vi "test-ltv-unicycle-controller-Test2.vi"() -> (3 "All tests passed":bool)   [LabVIEW 2019]
uses:
  <vilib>/Rock Robotics/WPI/ThirdParty/JAS_Junk/TrajLib/Trajectory_Library.lvlib
  <vilib>/Rock Robotics/WPI/ThirdParty/JAS_Junk/TrajLib/Enum/TRAJECTORY_SPLINE_TYPE_ENUM.ctl
  <vilib>/numeric/Random Number (Range) DBL.vi
  <vilib>/Rock Robotics/WPI/ThirdParty/JAS_Junk/TrajLib/TypeDef/TRANSLATION2D.ctl
  <vilib>/Rock Robotics/WPI/ThirdParty/JAS_Junk/TrajLib/TypeDef/ROTATION2D.ctl
  <vilib>/Rock Robotics/WPI/ThirdParty/JAS_Junk/TrajLib/TypeDef/POSE2D.ctl
  <vilib>/Rock Robotics/WPI/ThirdParty/JAS_Junk/TrajLib/TypeDef/TRAJ_STATE.ctl
  <vilib>/Rock Robotics/WPI/ThirdParty/JAS_Junk/TrajLib/TypeDef/TRAJECTORY.ctl
  <vilib>/Rock Robotics/WPI/ThirdParty/JAS_Junk/TrajLib/TypeDef/CHASSIS_SPEEDS.ctl
  <vilib>/Rock Robotics/WPI/ThirdParty/JAS_Junk/TrajLib/TypeDef/LTV_UNICYCLE_CONTROLLER.ctl
  <vilib>/Rock Robotics/WPI/ThirdParty/JAS_Junk/TrajLib/TypeDef/FUNCTION_GENERATOR_MATRIX.ctl
panel:
  in  "Use Rate Limit":bool=TRUE
  in  "Use Noise":bool
  out "Any Calc Error":bool
  out "At Reference":bool
  out "Waveform Graph":dbl[][](graph)
  out "Ctrl":T1={"States"=0, "Inputs"=0, "PoseError"={"TRANSLATION"={"X"=0.0, "Y"=0.0}, "ROTATION"={"VALUE"=0.0, "COS"=1.0, "SIN"=0.0}}, "PoseTolerance"={"TRANSLATION"={"X"=0.0, "Y"=0.0}, "ROTATION"={"VALUE"=0.0, "COS"=1.0, "SIN"=0.0}}, "Dt"=0.02, "Enabled"=FALSE, "LQR_K_Table"={"Table Xs"=[], "Table Ys"=[], "MinX"=0.0, "MaxX"=0.0, "ItemCount"=0, "Rows"=0, "Columns"=0}} {"PoseTolerance"."ROTATION"."SIN" format="%13.4f"; "PoseTolerance"."ROTATION"."COS" format="%13.4f"; "PoseTolerance"."ROTATION"."VALUE" format="%13.4f"; "PoseTolerance"."TRANSLATION"."Y" format="%14.3f"; "PoseTolerance"."TRANSLATION"."X" format="%14.3f"; "PoseError"."ROTATION"."SIN" format="%13.4f"; "PoseError"."ROTATION"."COS" format="%13.4f"; "PoseError"."ROTATION"."VALUE" format="%13.4f"; "PoseError"."TRANSLATION"."Y" format="%14.3f"; "PoseError"."TRANSLATION"."X" format="%14.3f"}
  out "ChassisSpeeds":T6 {"vOmega" format="%10.3f"; "vY" format="%10.3f"; "vX" format="%10.3f"}
  out "XY Graph":cluster{dbl[], dbl[]}[](graph)
  out "X":bool
  out "Y":bool
  out "Rot":bool
  out "TotalTime_Sec":dbl
  out "OutputTRAJ_STATE":T7={"TimeSeconds"=0.0, "Velocity"=0.0, "Acceleration"=0.0, "POSE"={"TRANSLATION"={"X"=0.0, "Y"=0.0}, "ROTATION"={"VALUE"=0.0, "COS"=1.0, "SIN"=0.0}}, "Curvature"=0.0} {"POSE"."ROTATION"."SIN" format="%13.4f"; "POSE"."ROTATION"."COS" format="%13.4f"; "POSE"."ROTATION"."VALUE" format="%13.4f"; "POSE"."TRANSLATION"."Y" format="%14.3f"; "POSE"."TRANSLATION"."X" format="%14.3f"}
  out "UpdatedPose":T2 {"ROTATION"."SIN" format="%13.4f"; "ROTATION"."COS" format="%13.4f"; "ROTATION"."VALUE" format="%13.4f"; "TRANSLATION"."Y" format="%14.3f"; "TRANSLATION"."X" format="%14.3f"}
  out "TrajStatePose":T2={"TRANSLATION"={"X"=0.0, "Y"=0.0}, "ROTATION"={"VALUE"=0.0, "COS"=1.0, "SIN"=0.0}} {"ROTATION"."SIN" format="%13.4f"; "ROTATION"."COS" format="%13.4f"; "ROTATION"."VALUE" format="%13.4f"; "TRANSLATION"."Y" format="%14.3f"; "TRANSLATION"."X" format="%14.3f"}
  out "Calc Error":bool
  out "Create\nError":bool
  out "TRAJECTORY":T8 {"States"."POSE"."ROTATION"."SIN" format="%13.4f"; "States"."POSE"."ROTATION"."COS" format="%13.4f"; "States"."POSE"."ROTATION"."VALUE" format="%13.4f"; "States"."POSE"."TRANSLATION"."Y" format="%14.3f"; "States"."POSE"."TRANSLATION"."X" format="%14.3f"; "TotalTImeSecs" format="%20.3f"}
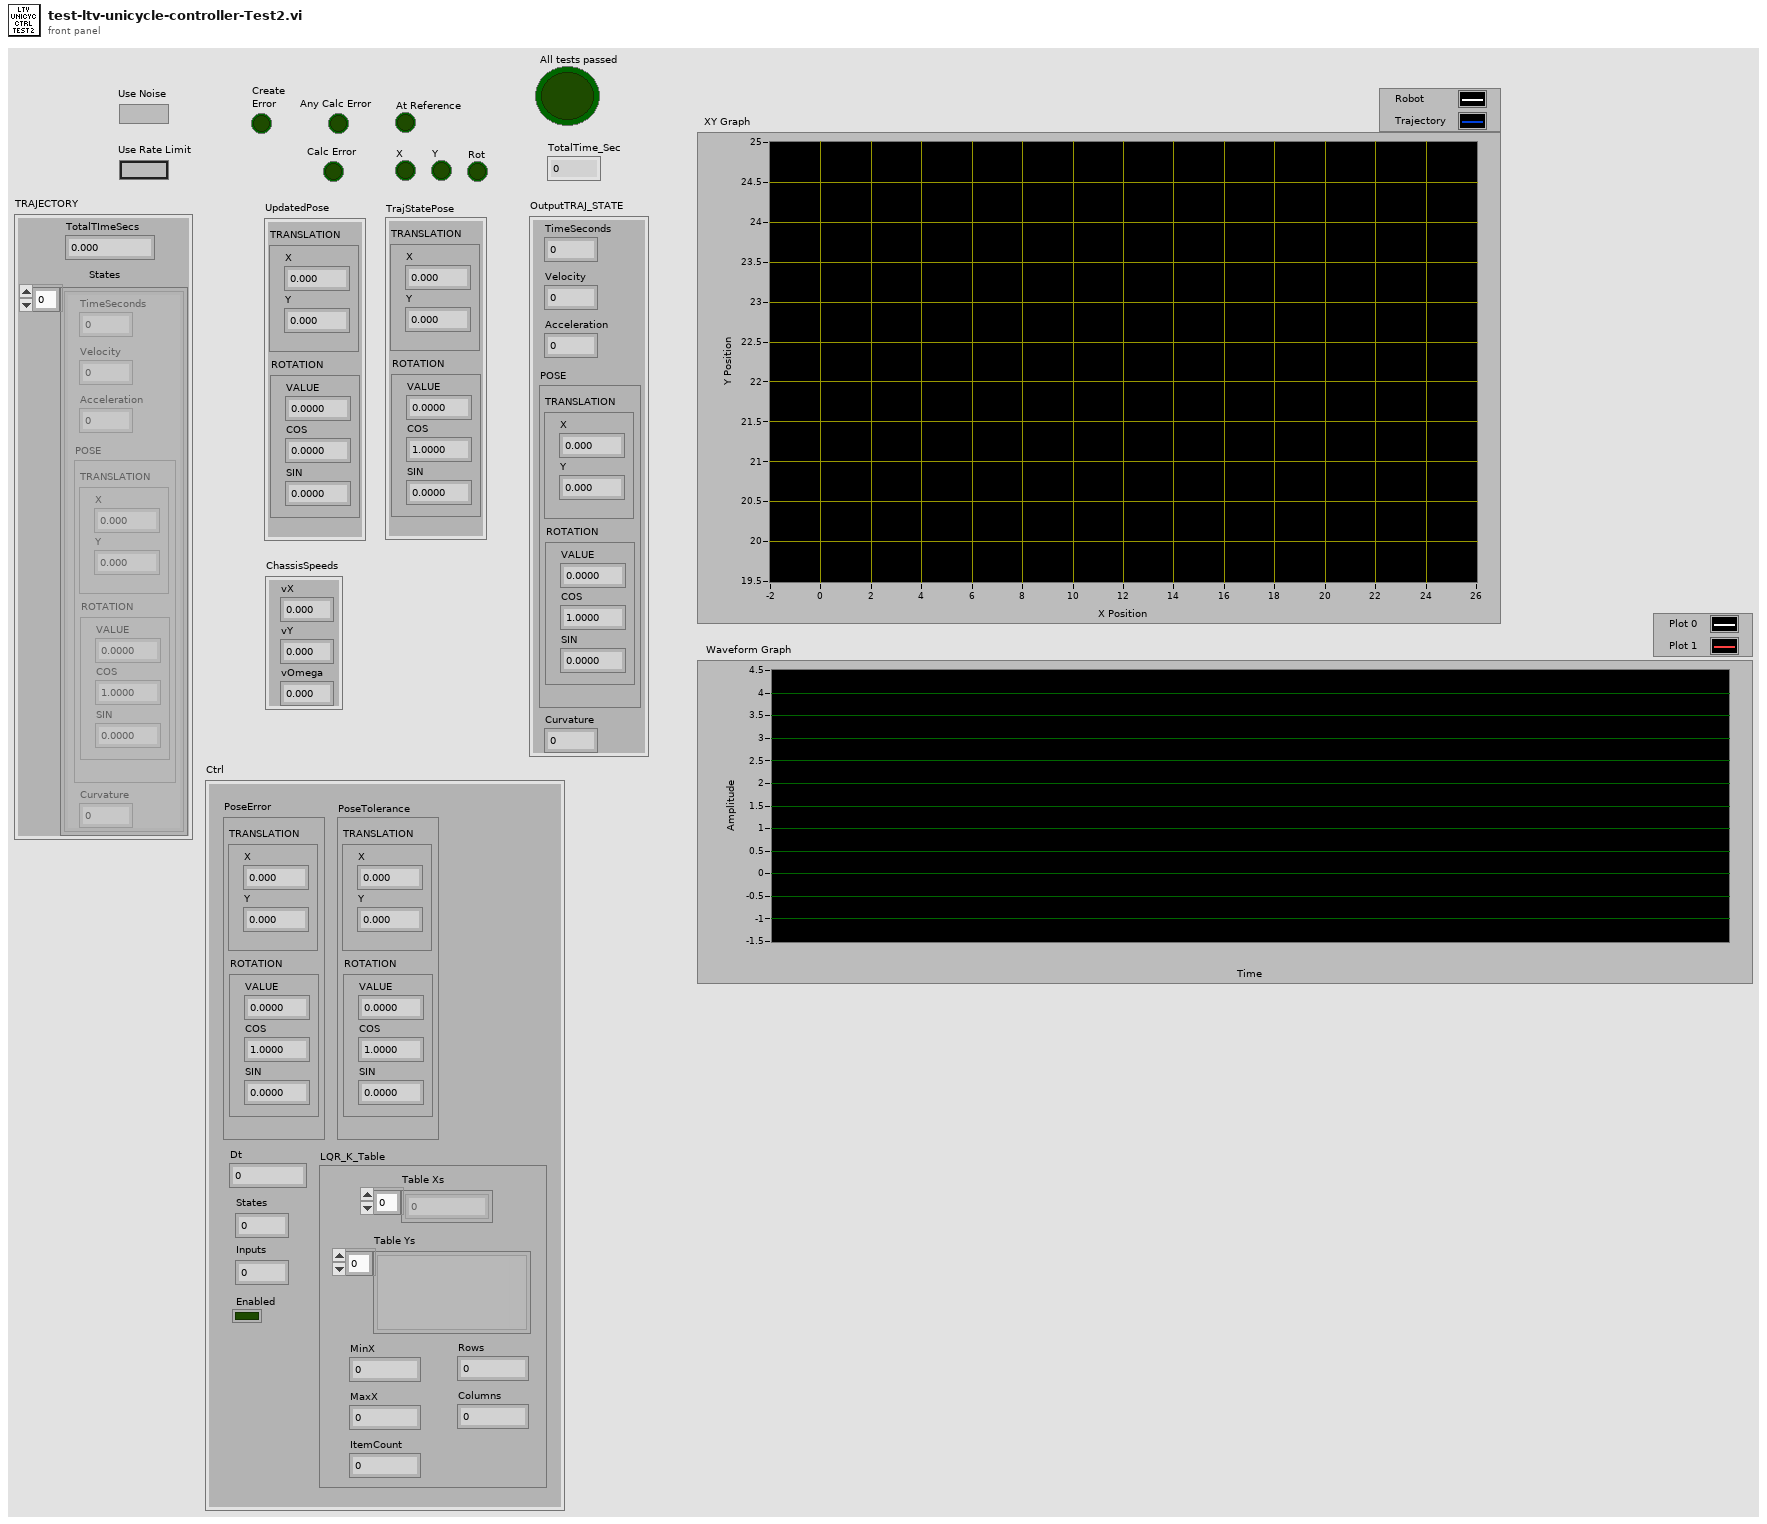
[diagram p1: front panel]
types:
  T1 = typedef "Trajectory_Library.lvlib/LTV_UNICYCLE_CONTROLLER.ctl" = cluster{"States":i32, "Inputs":i32, "PoseError":T2, "PoseTolerance":T2, "Dt":dbl, "Enabled":bool, "LQR_K_Table":T5}
  T2 = typedef "Trajectory_Library.lvlib/POSE2D.ctl" = cluster{"TRANSLATION":T3, "ROTATION":T4}
  T3 = typedef "Trajectory_Library.lvlib/TRANSLATION2D.ctl" = cluster{"X":dbl, "Y":dbl}
  T4 = typedef "Trajectory_Library.lvlib/ROTATION2D.ctl" = cluster{"VALUE":dbl, "COS":dbl, "SIN":dbl}
  T5 = typedef "Trajectory_Library.lvlib/FUNCTION_GENERATOR_MATRIX.ctl" = cluster{"Table Xs":dbl[], "Table Ys":variant[], "MinX":dbl, "MaxX":dbl, "ItemCount":i32, "Rows":i32, "Columns":i32}
  T6 = typedef "Trajectory_Library.lvlib/CHASSIS_SPEEDS.ctl" = cluster{"vX":dbl, "vY":dbl, "vOmega":dbl}
  T7 = typedef "Trajectory_Library.lvlib/TRAJ_STATE.ctl" = cluster{"TimeSeconds":dbl, "Velocity":dbl, "Acceleration":dbl, "POSE":T2, "Curvature":dbl}
  T8 = typedef "Trajectory_Library.lvlib/TRAJECTORY.ctl" = cluster{"TotalTImeSecs":dbl, "States":T7[]}
  T9 = typedef "Trajectory_Library.lvlib/TRAJECTORY_SPLINE_TYPE_ENUM.ctl" = enum16{"Cubic", "Cubic With Weights", "Quintic", "Quintic With Weights"}
  T10 = typedef "Trajectory_Library.lvlib/WEIGHTED_WAYPOINT.ctl" = cluster{"TRANSLATION":T3, "ROTATION":T4, "SCALAR":dbl}
  T11 = typedef "Trajectory_Library.lvlib/TRAJ_CONFIG.ctl" = cluster{"MaxVelocity":dbl, "Max Acceleration":dbl, "StartVelocity":dbl, "End Velocity":dbl, "Reversed":bool, "Constraints":variant[]}
  T12 = typedef "NI_Matrix.lvlib/RealMatrix.ctl" = dbl[][]
  T13 = typedef "Trajectory_Library.lvlib/TWIST2D.ctl" = cluster{"dX":dbl, "dY":dbl, "dTHETA":dbl}
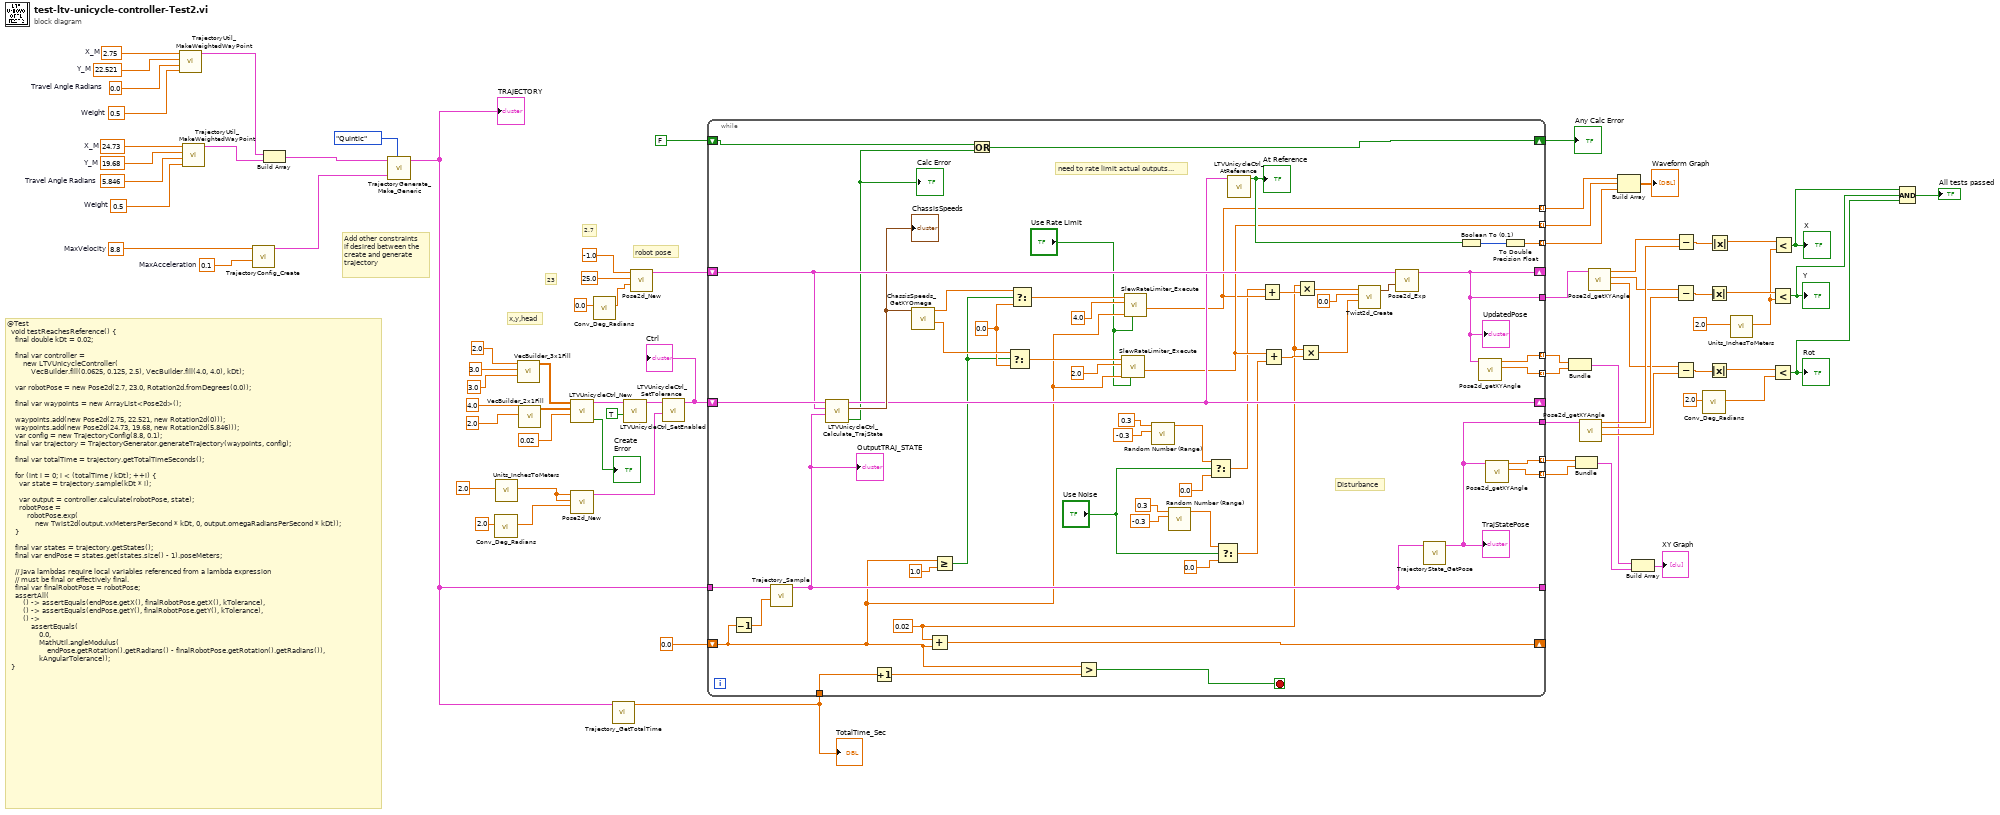
[diagram p0: block diagram]
diagram:
  w63 = 24.73  # X_M
  w62 = 19.68  # Y_M
  w50 = 5.846  # Travel Angle Radians
  w61 = 0.5  # Weight
  w60 = 2.75  # X_M
  w59 = 22.521  # Y_M
  w51 = 0.0  # Travel Angle Radians
  w58 = 0.5  # Weight
  w57 = 8.8  # MaxVelocity
  w56 = 0.1  # MaxAcceleration
  # "23"
  # "2.7"
  # "x,y,head"
  # "@Test\n  void testReachesReference() {\n    final double kDt = 0.02;\n\n    final var controller =\n        new LTVUnicycleController(\n            VecBuilder.fill(0.0625, 0.125, 2.5), VecBuilder.fill(4.0, 4.0), kDt);\n\n    var robotPose = new Pose2d(2.7, 23.0, Rotation2d.fromDegrees(0.0));\n\n    final var waypoints = new ArrayList<Pose2d>();\n\n    waypoints.add(new Pose2d(2.75, 22.521, new Rotation2d(0)));\n    waypoints.add(new Pose2d(24.73, 19.68, new Rotation2d(5.846)));\n    var config = new TrajectoryConfig(8.8, 0.1);\n    final var trajectory = TrajectoryGenerator.generateTrajectory(waypoints, config);\n\n    final var totalTime = trajectory.getTotalTimeSeconds();\n\n    for (int i = 0; i < (totalTime / kDt); ++i) {\n      var state = trajectory.sample(kDt * i);\n\n      var output = controller.calculate(robotPose, state);\n      robotPose =\n          robotPose.exp(\n              new Twist2d(output.vxMetersPerSecond * kDt, 0, output.omegaRadiansPerSecond * kDt));\n    }\n\n    final var states = trajectory.getStates();\n    final var endPose = states.get(states.size() - 1).poseMeters;\n\n    // Java lambdas require local variables referenced from a lambda expression\n    // must be final or effectively final.\n    final var finalRobotPose = robotPose;\n    assertAll(\n        () -> assertEquals(endPose.getX(), finalRobotPose.getX(), kTolerance),\n        () -> assertEquals(endPose.getY(), finalRobotPose.getY(), kTolerance),\n        () ->\n            assertEquals(\n                0.0,\n                MathUtil.angleModulus(\n                    endPose.getRotation().getRadians() - finalRobotPose.getRotation().getRadians()),\n                kAngularTolerance));\n  }"
  # "Add other constraints\nif desired between the\ncreate and generate\ntrajectory"
  # "robot pose"
  n1 = call <vilib>:"TrajectoryUtil_MakeWeightedWayPoint.vi"("Weight"=w58, "Travel Angle Radians"=w51, "Y_M"=w59, "X_M"=w60) -> ("WEIGHTED_WAYPOINT"=w52:T10)  [unwired: 7 in]
  n2 = call <vilib>:"TrajectoryUtil_MakeWeightedWayPoint.vi"("Weight"=w61, "Travel Angle Radians"=w50, "Y_M"=w62, "X_M"=w63) -> ("WEIGHTED_WAYPOINT"=w64:T10)  [unwired: 7 in]
  n3 = call <vilib>:"TrajectoryConfig_Create.vi"("MaxAcceleration"=w56, "MaxVelocity"=w57) -> ("TRAJECTORY_CONFIG"=w55:T11)  [unwired: 9 in]
  n4 = Build Array(w52, w64) -> (w53:T10[])
  n5 = call <vilib>:"TrajectoryGenerate_Make_Generic.vi"("Spline Type"=TRAJECTORY_SPLINE_TYPE_ENUM."Quintic", "traj_config"=w55, "WeightedWayPoints"=w53) -> ("TRAJECTORY"=w47:T8)  [unwired: 7 in, 1 out]
  "TRAJECTORY" <- w47
  n6 = call <vilib>:"Conv_Deg_Radians.vi"("Degress"=2.0) -> ("Radians"=w13:dbl)  [unwired: 10 in]
  n7 = call <vilib>:"Units_InchesToMeters.vi"("Inches"=2.0 ("x")) -> ("Meters"=w2:dbl)  [unwired: 10 in]
  n8 = call <vilib>:"VecBuilder_3x1Fill.vi"("R2"=3.0, "R1"=3.0, "R0"=2.0) -> ("output matrix"=w75:T12)  [unwired: 8 in]
  n9 = call <vilib>:"VecBuilder_2x1Fill.vi"("R1"=2.0, "R0"=4.0) -> ("output matrix"=w74:T12)  [unwired: 9 in]
  n10 = call <vilib>:"LTVUnicycleCtrl_New.vi"("dT"=0.02, "RELMS"=w74, "QELMS"=w75) -> ("Error"=→"Create\nError":bool, "LTV_UNICYCLE_CONTROLLER"=w21:T1)  [unwired: 7 in]
  n11 = call <vilib>:"Pose2d_New.vi"("Heading"=w13, "Y"=w2, "X"=w2) -> ("out POSe"=w12:T2)  [unwired: 8 in]
  n12 = call <vilib>:"Conv_Deg_Radians.vi"("Degress"=0.0) -> ("Radians"=w68:dbl)  [unwired: 10 in]
  n13 = call <vilib>:"Trajectory_GetTotalTime.vi"("TRAJECTORY"=w47) -> ("TotalTime_Sec"=w48:dbl)  [unwired: 10 in]
  "TotalTime_Sec" <- w48
  n14 = call <vilib>:"LTVUnicycleCtrl_SetEnabled.vi"("Enabled"=TRUE, "in LTV_UNICYCLE_CONTROLLER"=w21) -> ("out LTV_UNICYCLE_CONTROLLER"=w15:T1)  [unwired: 9 in]
  n15 = call <vilib>:"Pose2d_New.vi"("Heading"=w68, "Y"=25.0, "X"=-1.0) -> ("out POSe"=w46:T2)  [unwired: 8 in]
  n16 = call <vilib>:"LTVUnicycleCtrl_SetTolerance.vi"("Tolerance"=w12, "in LTV_UNICYCLE_CONTROLLER"=w15) -> ("out LTV_UNICYCLE_CONTROLLER"=w14:T1)  [unwired: 9 in]
  "Ctrl" <- w14
  n17 = while {
    shift-right: [w129] -> _
    shift-left: 0.0 -> [w80]
    tunnel: w48 -> [w82]
    tunnel: w47 -> [w128]
    shift-right: [w115] -> _
    shift-left: w46 -> [w126]
    shift-right: [w111] -> _
    shift-left: w14 -> [w127]
    tunnel: [w120] -> _
    tunnel: [w114] -> w44
    tunnel: [w119] -> w29 mode=indexing
    tunnel: [w118] -> w28 mode=indexing
    tunnel: [w117] -> w27 mode=indexing
    tunnel: [w116] -> w26 mode=indexing
    tunnel: [w115] -> w22
    tunnel: [w105] -> w19 mode=indexing
    tunnel: [w107] -> w17 mode=indexing
    tunnel: [w108] -> w11 mode=indexing
    shift-right: [w97] -> w5
    shift-left: FALSE -> [w99]
    stop <- w130 stop-if-true
    w84 = 0.0 ("f")
    w89 = 0.02 ("x")
    # "Disturbance"
    # "need to rate limit actual outputs..."
    n18 = Decrement(x=w80) -> (x-1=w79:dbl)
    n19 = call <vilib>:"Trajectory_Sample.vi"("Time"=w79, "InputTRAJECTORY"=w128) -> ("OutputTRAJ_STATE"=w120:T7)  [unwired: 9 in]
    "OutputTRAJ_STATE" <- w120
    n20 = call <vilib>:"LTVUnicycleCtrl_Calculate_TrajState.vi"("TRAJ_STATE"=w120, "CurrentPose"=w126, "in LTV_UNICYCLE_CONTROLLER"=w127) -> ("Error"=w98:bool, "ChassisSpeeds"=w124:T6, "out LTV_UNICYCLE_CONTROLLER"=w111:T1)  [unwired: 6 in]
    "Calc Error" <- w98
    "ChassisSpeeds" <- w124
    n21 = Increment(x=w82) -> (x+1=w81:dbl)
    n22 = call <vilib>:"ChassisSpeeds_GetXYOmega.vi"("CHASSIS"=w124) -> ("vAngular"=w85:dbl, "vX"=w86:dbl)  [unwired: 8 in, 1 out]
    n23 = Add(x=w89, y=w80) -> (x+y=w129:dbl)
    n24 = Greater Or Equal?(x=w80, y=1.0) -> (x >= y?=w83:bool)
    n25 = Or(x=w99, y=w98) -> (x .or. y?=w97:bool)
    n26 = Select(t=w85, s=w83, f=w84) -> (s? t:f=w88:dbl)
    n27 = Select(t=w86, s=w83, f=w84) -> (s? t:f=w87:dbl)
    n28 = Greater?(x=w80, y=w81) -> (0:w130:bool)
    n29 = call <vilib>:"SlewRateLimiter_Execute.vi"("Enable"="Use Rate Limit", "Time"=w80, "PositiveRate"=2.0 ("Rate"), "Input"=w88) -> ("Output"=w107:dbl)  [unwired: 6 in, 1 out]
    n30 = call <vilib>:"SlewRateLimiter_Execute.vi"("Enable"="Use Rate Limit", "Time"=w80, "PositiveRate"=4.0 ("Rate"), "Input"=w87) -> ("Output"=w105:dbl)  [unwired: 6 in, 1 out]
    n31 = call-poly <vilib>:"Random Number (Range).vi"("lower bound (0)"=-0.3, "upper bound (100)"=0.3) -> ("number"=w94:dbl)  [unwired: 9 in]
    n32 = call-poly <vilib>:"Random Number (Range).vi"("lower bound (0)"=-0.3, "upper bound (100)"=0.3) -> ("number"=w91:dbl)  [unwired: 9 in]
    n33 = Select(t=w94, s="Use Noise", f=0.0) -> (s? t:f=w96:dbl)
    n34 = Select(t=w91, s="Use Noise", f=0.0) -> (s? t:f=w92:dbl)
    n35 = call <vilib>:"LTVUnicycleCtrl_AtReference.vi"("LTV_UNICYCLE_CONTROLLER"=w111) -> ("At Reference"=w110:bool)  [unwired: 10 in]
    "At Reference" <- w110
    n36 = Add(x=w96, y=w105) -> (x+y=w104:dbl)
    n37 = Add(x=w107, y=w92) -> (x+y=w106:dbl)
    n38 = Multiply(x=w89, y=w104) -> (x*y=w123:dbl)
    n39 = Multiply(x=w89, y=w106) -> (x*y=w121:dbl)
    n40 = call <vilib>:"Twist2d_Create.vi"("dTHETA"=w121, "dY"=0.0, "dX"=w123) -> ("TWIST"=w125:T13)  [unwired: 8 in]
    n41 = call <vilib>:"Pose2d_Exp.vi"("TWIST"=w125, "POSE"=w126) -> ("UpdatedPose"=w115:T2)  [unwired: 9 in]
    "UpdatedPose" <- w115
    n42 = call <vilib>:"TrajectoryState_GetPose.vi"("TRAJ_STATE"=w120) -> ("TrajStatePose"=w114:T2)  [unwired: 10 in]
    "TrajStatePose" <- w114
    n43 = Boolean To (0,1)(Boolean=w110) -> (0, 1=w109:i16)
    n44 = call <vilib>:"Pose2d_getXYAngle.vi"("in POSE"=w115) -> ("Y"=w118:dbl, "X"=w119:dbl)  [unwired: 8 in, 1 out]
    n45 = call <vilib>:"Pose2d_getXYAngle.vi"("in POSE"=w114) -> ("Y"=w116:dbl, "X"=w117:dbl)  [unwired: 8 in, 1 out]
    n46 = To Double Precision Float(number=w109) -> (double precision float=w108:dbl)
  }
  "Any Calc Error" <- w5
  n47 = Bundle(w29, w28) -> (w25:cluster{dbl[], dbl[]})  [unwired: 1 in]
  n48 = Bundle(w27, w26) -> (w24:cluster{dbl[], dbl[]})  [unwired: 1 in]
  n49 = call <vilib>:"Pose2d_getXYAngle.vi"("in POSE"=w44) -> ("Angle"=w32:dbl, "Y"=w34:dbl, "X"=w40:dbl)  [unwired: 8 in]
  n50 = call <vilib>:"Pose2d_getXYAngle.vi"("in POSE"=w22) -> ("Angle"=w33:dbl, "Y"=w35:dbl, "X"=w41:dbl)  [unwired: 8 in]
  n51 = Build Array(w19, w17, w11) -> (→"Waveform Graph":dbl[][])
  n52 = Build Array(w25, w24) -> (→"XY Graph":cluster{dbl[], dbl[]}[])
  n53 = Subtract(x=w35, y=w34) -> (x-y=w38:dbl)
  n54 = Subtract(x=w33, y=w32) -> (x-y=w36:dbl)
  n55 = Subtract(x=w41, y=w40) -> (x-y=w42:dbl)
  n56 = call <vilib>:"Conv_Deg_Radians.vi"("Degress"=2.0) -> ("Radians"=w30:dbl)  [unwired: 10 in]
  n57 = Absolute Value(x=w38) -> (abs(x)=w39:dbl)
  n58 = Absolute Value(x=w36) -> (abs(x)=w37:dbl)
  n59 = Absolute Value(x=w42) -> (abs(x)=w43:dbl)
  n60 = call <vilib>:"Units_InchesToMeters.vi"("Inches"=2.0 ("x")) -> ("Meters"=w4:dbl)  [unwired: 10 in]
  n61 = Less?(x=w39, y=w4) -> (x < y?=w8:bool)
  "Y" <- w8
  n62 = Less?(x=w37, y=w30) -> (x < y?=w7:bool)
  "Rot" <- w7
  n63 = Less?(x=w43, y=w4) -> (x < y?=w9:bool)
  "X" <- w9
  n64 = Compound Arithmetic op=AND(w9, w8, w7) -> (→"All tests passed":bool)
